vi "Compile NTeethMMissing.vi"(7 "Custom Device Ref":T1 format="%.0x", 8 "error in (no error)":errorcluster, 10 "Channel Descriptors in":T2, 11 "N Teeth M Missing refs":T1[](array[typedef]) format="%.0x") -> (0 "error out":errorcluster, 2 "Channel Descriptors out":T2, 4 "N Teeth M Missing":T9[](array[typedef]))   [LabVIEW 2011, in "Engine Sim System Explorer.lvlib"]
uses:
  Engine Sim System Explorer.lvlib
  Shared/NTeethConfig.ctl
  <vilib>/NI Veristand/Custom Device API/Custom Device Item Ref.ctl
  Shared/Channel Descriptors.ctl
  Shared/FPGA Write Descriptor.ctl
  Shared/InputChannelTypes.ctl
  <vilib>/rvi/DataTransferAndStorage/Container/Common/niFpgaDataTypeControl.ctl
  Shared/FPGA Read Descriptor.ctl
  Shared/OutputChannelTypes.ctl
  Shared/Status Chan Descriptor.ctl
  TypeDefs/NTeethSettings.ctl
  Shared/Engine Simulation Global.vi
  <vilib>/NI Veristand/Custom Device API/Get Item Property (Boolean).vi
  <vilib>/NI Veristand/Custom Device API/Get Item Property (Variant).vi
  <vilib>/NI Veristand/Custom Device API/Custom Device API.lvlib
  <userlib>/AES/RT/AES RT.lvlib
  Engine Simulation Shared.lvlib
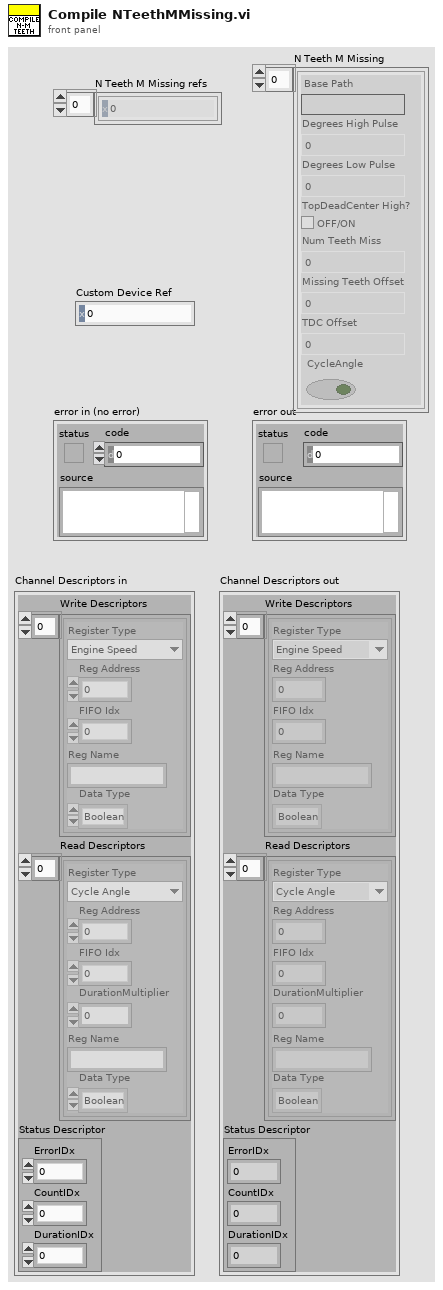
[diagram p1: front panel]
types:
  T1 = typedef "Custom Device API.lvlib/Custom Device Item Ref.ctl" = u64
  T2 = typedef "Engine Simulation Shared.lvlib/Channel Descriptors.ctl" = cluster{"Write Descriptors":T3[], "Read Descriptors":T6[], "Status Descriptor":T8}
  T3 = typedef "Engine Simulation Shared.lvlib/FPGA Write Descriptor.ctl" = cluster{"Register Type":T4, "Reg Address":u32, "FIFO Idx":i32, "Reg Name":string, "Data Type":T5}
  T4 = typedef "Engine Simulation Shared.lvlib/InputChannelTypes.ctl" = enum16{"Engine Speed", "Offset"}
  T5 = typedef "niFpgaDataTypeControl.ctl" = enum32{"Boolean", "I8", "I16", "I32", "I64", "U8", "U16", "U32", "U64", "FXP", "CustomControl"}
  T6 = typedef "Engine Simulation Shared.lvlib/FPGA Read Descriptor.ctl" = cluster{"Register Type":T7, "Reg Address":u32, "FIFO Idx":i32, "DurationMultiplier":dbl, "Reg Name":string, "Data Type":T5}
  T7 = typedef "Engine Simulation Shared.lvlib/OutputChannelTypes.ctl" = enum16{"Cycle Angle", "Crank Angle", "Time Duration", "Angle Duration", "Start Angle", "End Angle"}
  T8 = typedef "Engine Simulation Shared.lvlib/Status Chan Descriptor.ctl" = cluster{"ErrorIDx":i32, "CountIDx":i32, "DurationIDx":i32}
  T9 = typedef "Engine Simulation Shared.lvlib/NTeethConfig.ctl" = cluster{"Base Path":string, "Degrees High Pulse":u64, "Degrees Low Pulse":u64, "TopDeadCenter High?":bool, "Num Teeth Miss":u8, "Missing Teeth Offset":u64, "TDC Offset":u64, "CycleAngle":bool}
  T10 = enum16{"Beginning of Tooth", "Middle of Tooth", "Beginning of Gap", "Middle of Gap"}
  T11 = typedef "Engine Sim System Explorer.lvlib/NTeethSettings.ctl" = cluster{"Tooth/Gap Duty Cycle":dbl, "Number of Teeth":u8, "Number Missing Teeth":u8, "Location Missing Teeth":dbl, "TDC Configuration":enum16{"Beginning of Tooth", "Middle of Tooth", "Beginning of Gap", "Middle of Gap"}}
  T12 = typedef "Custom Device API.lvlib/Custom Device Item Info.ctl" = cluster{"Name":string, "Is Channel":bool, "GUID":string}
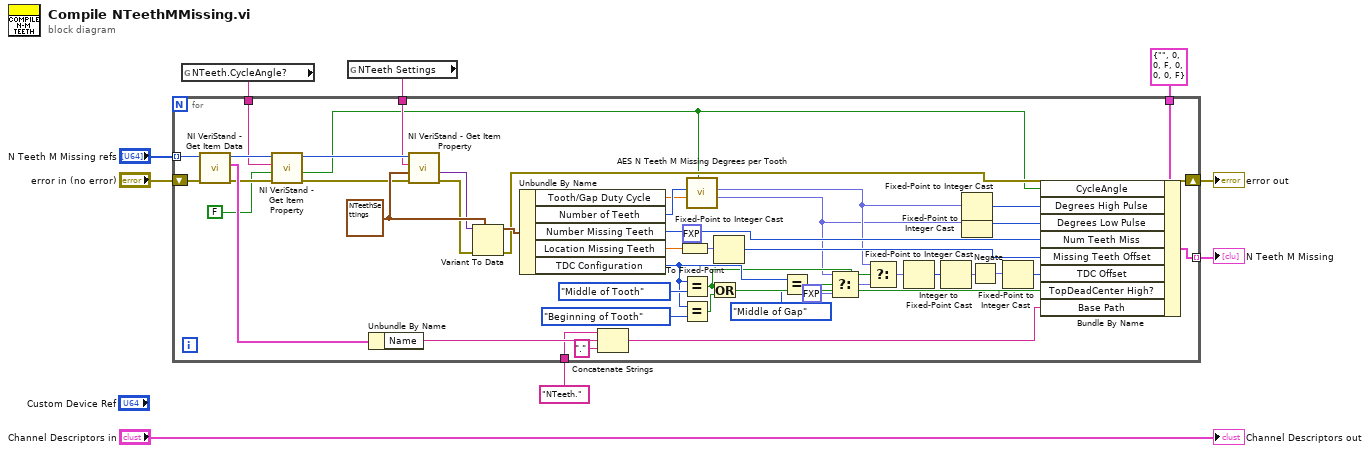
[diagram p0: block diagram]
diagram:
  n1 = global read "Engine Simulation Global.vi" "NTeeth.CycleAngle?"() -> (w8:string)
  n2 = global read "Engine Simulation Global.vi" "NTeeth Settings"() -> (w9:string)
  n3 = for {
    shift-right: [w43] -> w6
    shift-left: "error in (no error)" -> [w57]
    tunnel: "N Teeth M Missing refs" -> [w56] mode=indexing
    tunnel: T9 {"Base Path"="", "Degrees High Pulse"=0, "Degrees Low Pulse"=0, "TopDeadCenter High?"=FALSE, "Num Teeth Miss"=0, "Missing Teeth Offset"=0, "TDC Offset"=0, "CycleAngle"=FALSE} ("NTeeth Config") -> [w42]
    tunnel: [w36] -> w5 mode=indexing
    tunnel: "NTeeth." ("string") -> [w33]
    tunnel: w8 -> [w12]
    tunnel: w9 -> [w11]
    w55 = T11 {"Tooth/Gap Duty Cycle"=50.0, "Number of Teeth"=60, "Number Missing Teeth"=2, "Location Missing Teeth"=300.0, "TDC Configuration"=enum."Beginning of Tooth"} ("output cluster")
    n4 = call <vilib>:"NI VeriStand - Get Item Data.vi"("error in (no error)"=w57, "Item Ref in"=w56) -> ("error out"=w20:errorcluster, "Item Info"=w51:T12, "Item Ref out"=w19:T1)  [unwired: 6 in, 1 out]
    n5 = call-poly <vilib>:"NI VeriStand - Get Item Property.vi"("error in (no error)"=w20, "Default Value"=FALSE, "Property Name"=w12, "Item Ref in"=w19) -> ("error out"=w17:errorcluster, "Value"=w10:bool, "Item Ref out"=w18:T1)  [unwired: 4 in, 1 out]
    n6 = Unbundle By Name(w51) -> ("Name"=w35:string)
    n7 = call-poly <vilib>:"NI VeriStand - Get Item Property.vi"("error in (no error)"=w17, "Default Value"=w55, "Property Name"=w11, "Item Ref in"=w18) -> ("error out"=w53:errorcluster, "Value"=w52:variant)  [unwired: 4 in, 2 out]
    n8 = Variant To Data(error in=w53, type=w55, Variant=w52) -> (data=w54:T11, error out=w43:errorcluster)
    n9 = Unbundle By Name(w54) -> ("Tooth/Gap Duty Cycle"=w49:dbl, "Number of Teeth"=w50:u8, "Number Missing Teeth"=w39:u8, "Location Missing Teeth"=w45:dbl, "TDC Configuration"=w24:T10)
    n10 = Concatenate Strings(w33, w35, "." ("string")) -> (w32:string)
    n11 = To Fixed-Point(fixed-point type=fxp<+,61,10> 0.0 ("NTeeth.Crank.Missing Teeth Offset"), number=w45) -> (fixed-point=w37:fxp<+,61,10>)
    n12 = Equal?(x=w24, y=T10."Middle of Tooth") -> (x = y?=w23:bool)
    n13 = Equal?(x=w24, y=T10."Beginning of Tooth") -> (x = y?=w46:bool)
    n14 = call <userlib>:"AES N Teeth M Missing Degrees per Tooth.vi"("NTeeth.Use Cycle? (F)"=w10, "Crank.Teeth Duty Cycle"=w49, "NTeeth.Num Teeth"=w50) -> ("NTeeth.Degrees Low Pulse"=w13:fxp<+,60,9>, "NTeeth.Degrees High Pulse"=w14:fxp<+,60,9>)  [unwired: 7 in]
    n15 = Or(x=w23, y=w46) -> (x .or. y?=w31:bool)
    n16 = Fixed-Point to Integer Cast(1:w37) -> (0:w38:u64)
    n17 = Equal?(x=w24, y=T10."Middle of Gap") -> (x = y?=w25:bool)
    n18 = Select(t=w13, s=w25, f=fxp<+,58,7> 0.0 ("NTeeth.Degrees Low Pulse")) -> (s? t:f=w28:fxp<+,60,9>)
    n19 = Select(t=w14, s=w23, f=w28) -> (s? t:f=w27:fxp<+,60,9>)
    n20 = Fixed-Point to Integer Cast(1:w27) -> (0:w30:u64)
    n21 = Integer to Fixed-Point Cast(integer=w30) -> (fixed-point=w29:fxp<+,60,8>)  [unwired: 1 in]
    n22 = Fixed-Point to Integer Cast(1:w14) -> (0:w41:u64)
    n23 = Fixed-Point to Integer Cast(1:w13) -> (0:w40:u64)
    n24 = Negate(x=w29) -> (-x=w22:fxp<+/-,61,10>)
    n25 = Fixed-Point to Integer Cast(1:w22) -> (0:w21:i64)
    n26 = Bundle By Name(cluster=w42, "CycleAngle"=w10, "Degrees High Pulse"=w41, "Degrees Low Pulse"=w40, "Num Teeth Miss"=w39, "Missing Teeth Offset"=w38, "TDC Offset"=w21, "TopDeadCenter High?"=w31, "Base Path"=w32) -> (w36:T9)
  }
  "error out" <- w6
  "N Teeth M Missing" <- w5
  "Channel Descriptors out" <- "Channel Descriptors in"
